vi "Actor Core.vi"(8 "error in":errorcluster, 11 "Agilent DSO-X 3032A in":refnum<class "Agilent DSO-X 3032A.lvclass">) -> (0 "error out":errorcluster, 3 "Actor out":refnum<class "Actor.lvclass">)   [LabVIEW 2014, in "Agilent DSO-X 3032A.lvclass"]
doc: "(<B>Filename</B>: Actor Framework.lvlib:Actor.lvclass:Actor Core.vi)\n\nReceives messages to the actor, reacts to them, and initiates any error handling that may shut the actor down.\n\nDescendant classes may override this VI to append parallel tasks for the actor to complete while it handles messages. Overrides use the Call Parent Method node."
uses:
  Agilent DSO-X 3032A.lvclass
  <vilib>/ActorFramework/Actor/Actor.lvclass
  Framework/Model/Data/Data1D/Data1D.lvclass
  Channel Settings.ctl
  Agilent DSO-X 3032A.lvclass/Agilent DSO-X 3032A.ctl
  <vilib>/ActorFramework/Actor/Actor.lvclass/Actor.ctl
  <vilib>/ActorFramework/Message Enqueuer/Message Enqueuer.lvclass/Message Enqueuer.ctl
  Framework/Interfaces/Pipelined Actor/Pipelined Actor Messages/Do Main Action Msg/Do Main Action Msg.lvclass/Do Main Action Msg.ctl
  Agilent DSO-X 3032A Messages/Write Instrument Handle Msg/Write Instrument Handle Msg.lvclass/Write Instrument Handle Msg.ctl
  Agilent DSO-X 3032A Messages/Read Config From Device Msg/Read Config From Device Msg.lvclass/Read Config From Device Msg.ctl
  Agilent DSO-X 3032A Messages/Write Timeout Msg/Write Timeout Msg.lvclass/Write Timeout Msg.ctl
  Agilent DSO-X 3032A Messages/Write Settings Msg/Write Settings Msg.lvclass/Write Settings Msg.ctl
  Agilent DSO-X 3032A Messages/Write CurrentChannel Msg/Write CurrentChannel Msg.lvclass/Write CurrentChannel Msg.ctl
  <vilib>/ActorFramework/Message Enqueuer/Init from Existing Queue.vi
  <vilib>/ActorFramework/Message Enqueuer/Enqueue.vi
  <vilib>/ActorFramework/Message Priority Queue/Priority Enqueue.vi
  <vilib>/ActorFramework/Message Enqueuer/Message Enqueuer.lvclass
  Framework/Model/Data/AbstractData/AbstractData.lvclass
  Framework/Interfaces/Pipelined Actor/Pipelined Actor Messages/Do Main Action Msg/Do Main Action Msg.lvclass
  Framework/Hardware/Device/Device Messages/Disconnect Msg/Disconnect Msg.lvclass
  Agilent DSO-X 3032A Messages/Write Instrument Handle Msg/Write Instrument Handle Msg.lvclass
  Agilent DSO-X 3032A Messages/Read Config From Device Msg/Read Config From Device Msg.lvclass
  Agilent DSO-X 3032A Messages/Write Timeout Msg/Write Timeout Msg.lvclass
  Agilent DSO-X 3032A Messages/Write Settings Msg/Write Settings Msg.lvclass
  Agilent DSO-X 3032A Messages/Write CurrentChannel Msg/Write CurrentChannel Msg.lvclass
  Framework/Hardware/ReadoutDevice/ReadoutDevice.lvclass
  Framework/Interfaces/Viewable Actor/Viewable Actor.lvclass
  Framework/Interfaces/Observable Actor/Observable Actor.lvclass
panel:
  in  "Channel":string(combo)="CHAN1"
  in  "Timeout, ms":i32=1000000
  in  "Channel Settings":T1={"Dt"=0.002, "#samples"=10000, "t0"=0.0} {"Dt" format="%.2e"}
  in  "Path":path
  out "isReading":bool
  out "Latest Data":refnum<class "Data1D.lvclass">
  in  "Save":bool
  in  "Resource name":refnum<k15>="AGILENT"
  in  "Disconnect":bool
  in  "Connect":bool
  in  "Read Conf":bool
  out "Stop":bool=TRUE
  in  "Read":bool
  out "Preview Graph":waveform(dbl)(graph)
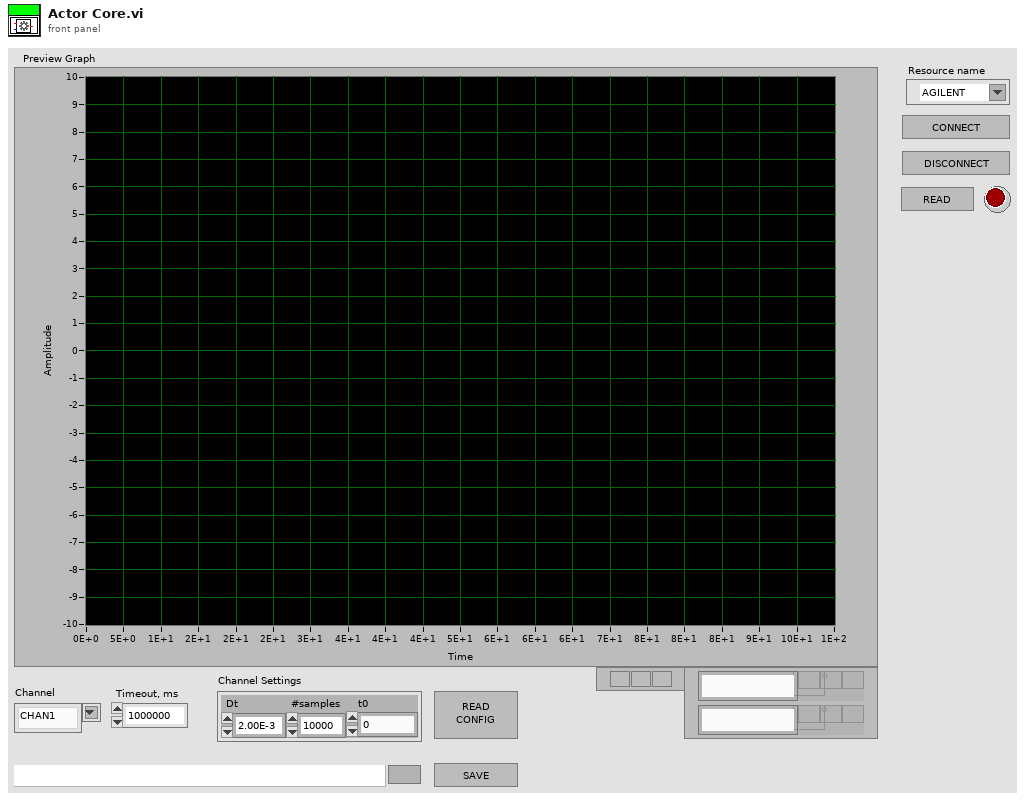
[diagram p1: front panel]
types:
  T1 = typedef "Agilent DSO-X 3032A.lvclass/Channel Settings.ctl" = cluster{"Dt":dbl, "#samples":i32, "t0":dbl}
  T2 = typedef "Observable Actor.lvlib/Observable Actor.lvclass/Observer.ctl" = refnum<queue>
  T3 = enum16{"open", "replace", "create", "open or create", "replace or create", "replace or create with confirmation"}
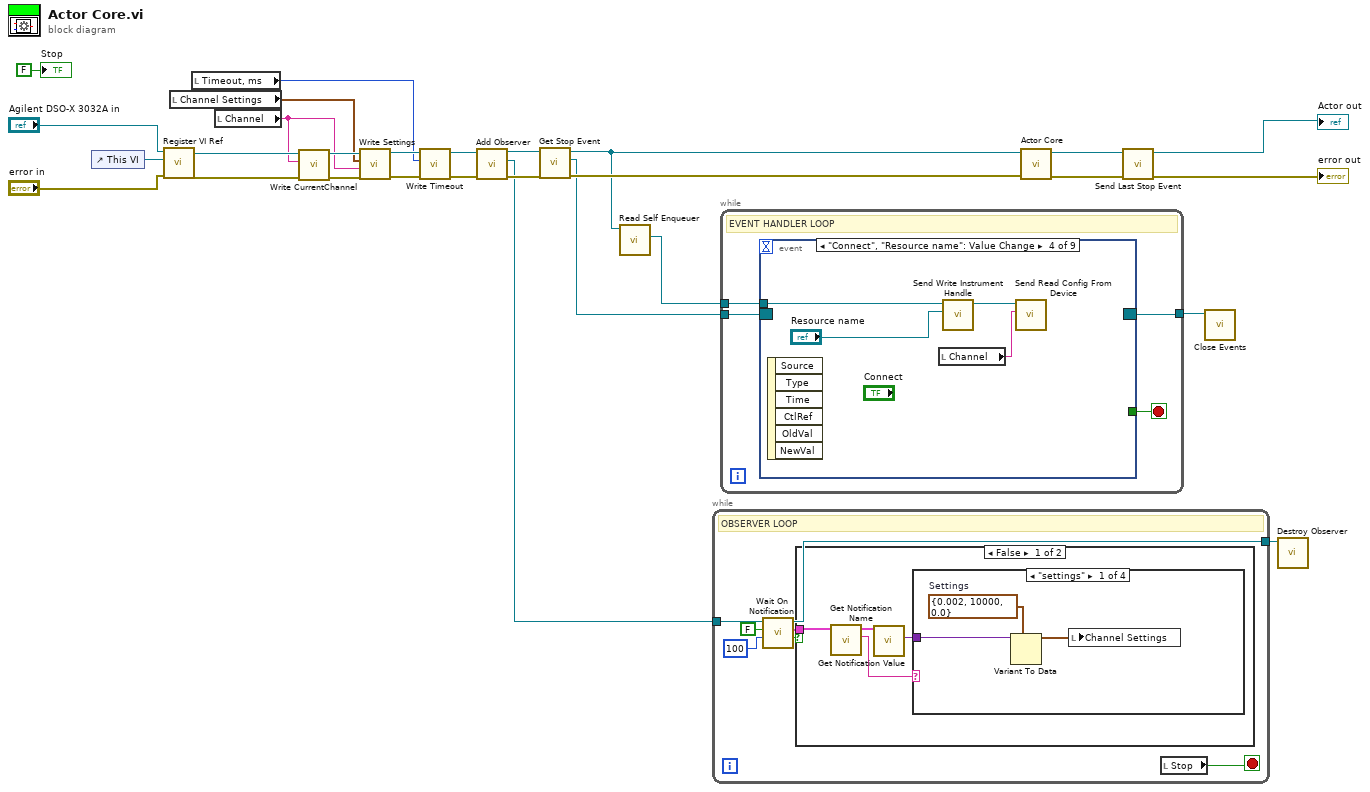
[diagram p0: block diagram]
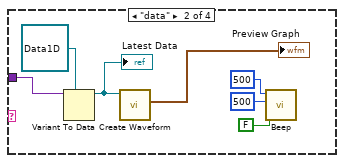
[diagram p2: hidden frame]
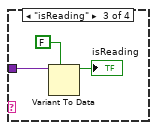
[diagram p3: hidden frame]
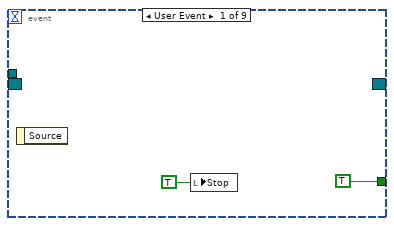
[diagram p6: hidden frame]
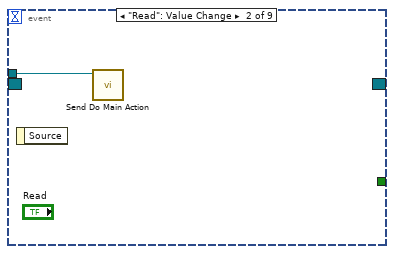
[diagram p7: hidden frame]
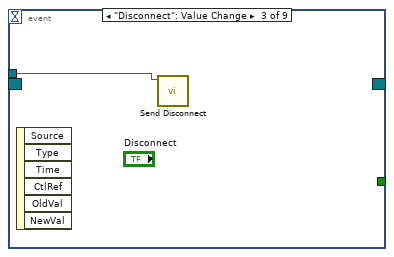
[diagram p8: hidden frame]
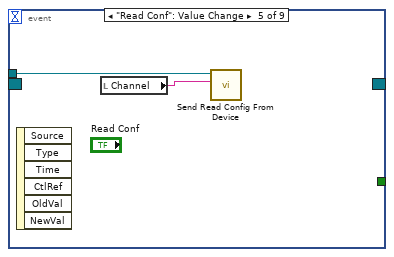
[diagram p9: hidden frame]
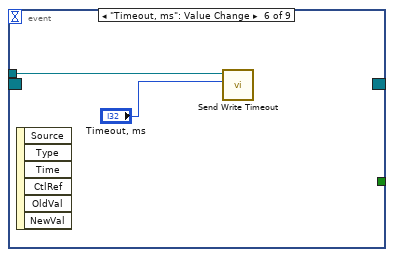
[diagram p10: hidden frame]
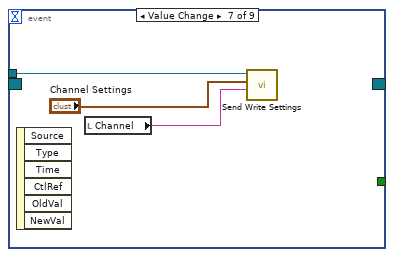
[diagram p11: hidden frame]
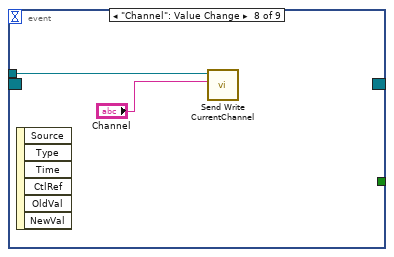
[diagram p12: hidden frame]
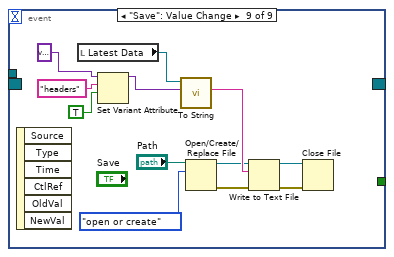
[diagram p13: hidden frame]
diagram:
  n1 = control-ref of="This VI"() -> (w27:refnum<vi>)
  n2 = call "Register VI Ref.vi"("error in (no error)"="error in", "VI ref"=w27, "Viewable Actor in"="Agilent DSO-X 3032A in") -> ("error out"=w10:errorcluster, "Viewable Actor out"=w11:refnum<class "Agilent DSO-X 3032A.lvclass">)  [unwired: 7 in]
  n3 = local read "Channel Settings"() -> (w7:T1)
  n4 = local read "Timeout, ms"() -> (w1:i32)
  n5 = local read "Channel"() -> (w8:string)
  n6 = call "Write CurrentChannel.vi"("error in (no error)"=w10, "CurrentChannel"=w8, "Agilent DSO-X 3032A in"=w11) -> ("error out"=w9:errorcluster, "Agilent DSO-X 3032A out"=w12:refnum<class "Agilent DSO-X 3032A.lvclass">)  [unwired: 7 in]
  n7 = call "Write Settings.vi"("error in (no error)"=w9, "Channel"=w8, "Settings"=w7, "Agilent DSO-X 3032A in"=w12) -> ("error out"=w4:errorcluster, "Agilent DSO-X 3032A out"=w5:refnum<class "Agilent DSO-X 3032A.lvclass">)  [unwired: 6 in]
  n8 = call "Write Timeout.vi"("error in (no error)"=w4, "Timeout"=w1, "Agilent DSO-X 3032A in"=w5) -> ("error out"=w3:errorcluster, "Agilent DSO-X 3032A out"=w2:refnum<class "Agilent DSO-X 3032A.lvclass">)  [unwired: 7 in]
  n9 = call-dynamic "Add Observer.vi"("error in (no error)"=w3, "Observable Actor in"=w2) -> ("error out"=w26:errorcluster, "new observer"=w24:T2, "Observable Actor out"=w23:refnum<class "Agilent DSO-X 3032A.lvclass">)  [unwired: 7 in]
  n10 = call-dynamic "Get Stop Event.vi"("error in (no error)"=w26, "Observable Actor in"=w23) -> ("error out"=w22:errorcluster, "Events"=w21:refnum<event-registration>, "Observable Actor out"=w13:refnum<class "Agilent DSO-X 3032A.lvclass">)  [unwired: 7 in]
  n11 = call <vilib>:"Read Self Enqueuer.vi"("Actor"=w13) -> ("Self Enqueuer"=w25:refnum<class "Message Enqueuer.lvclass">)  [unwired: 10 in]
  n12 = while {
    tunnel: w24 -> [w30]
    tunnel: [w29] -> w17
    stop <- w35 stop-if-true
    # "OBSERVER LOOP"
    n13 = call "Wait On Notification.vi"("timeout in ms (-1)"=100, "ignore previous (F)"=FALSE, "observer in"=w30) -> ("timed out?"=w31:bool, "notification"=w32:cluster{"value":variant, "name":string}, "observer out"=w29:T2)  [unwired: 5 in, 1 out]
    n14 = case shown="False" w31 {
      tunnel: w32 -> [w38 _]
      frame False {
        n15 = call "Get Notification Name.vi"("notification in"=w38) -> ("name"=w36:string, "notification out"=w37:cluster{"value":variant, "name":string})  [unwired: 9 in]
        n16 = call "Get Notification Value.vi"("notification in"=w37) -> ("data"=w39:variant)  [unwired: 7 in, 1 out]
        n17 = case shown="\"settings\"" w36 {
          tunnel: w39 -> [w42 w49 w51 _]
          frame "settings" {
            w41 = T1 {"Dt"=0.002, "#samples"=10000, "t0"=0.0}  # Settings
            n18 = Variant To Data(type=w41, Variant=w42) -> (data=w40:T1)  [unwired: 1 in, 1 out]
            n19 = local write "Channel Settings"(w40) -> ()
          }
          frame "data" {
            n20 = Variant To Data(type=refnum<class "Data1D.lvclass"> refnum ("Data1D in"), Variant=w49) -> (data=w47:refnum<class "Data1D.lvclass">)  [unwired: 1 in, 1 out]
            "Latest Data" <- w47
            n21 = call "Create Waveform.vi"("Data1D in"=w47) -> ("Waveform"=→"Preview Graph":waveform(dbl))  [unwired: 8 in, 2 out]
            n22 = call <vilib>:"Beep.vi"("use system alert? (T)"=FALSE, "duration (msec)"=u32 500, "frequency (Hz)"=u32 500) -> ()  [unwired: 9 in]
          }
          frame "isReading" {
            n23 = Variant To Data(type=FALSE, Variant=w51) -> (data=→"isReading":bool)  [unwired: 1 in, 1 out]
          }
          frame Default {
          }
        }
      }
      frame True {
      }
    }
    n24 = local read "Stop"() -> (w35:bool)
  }
  n25 = while {
    tunnel: w21 -> [w56]
    tunnel: w25 -> [w55]
    tunnel: [w54] -> w20
    stop <- w53 stop-if-true
    # "EVENT HANDLER LOOP"
    n26 = event shown="[3] \"Connect\", \"Resource name\": Value Change" {
      selector: w56 -> [_ _ _ _ _ _ _ _ _]
      dyn-events: [_ _ _ _ _ _ _ _ _] -> w54
      timeout: _ -> [_ _ _ _ _ _ _ _ _]
      tunnel: w55 -> [_ w59 w60 w64 w66 w68 w71 w73 _]
      tunnel: [TRUE _ _ _ _ _ _ _ _] -> w53
      event User Event {
        n27 = event-data() -> ()  [unwired: 1 in, 1 out]
        n28 = local write "Stop"(TRUE ("Stop")) -> ()
      }
      event "Read": Value Change {
        n29 = event-data() -> ()  [unwired: 1 in, 1 out]
        n30 = call "Send Do Main Action.vi"("Message Enqueuer"=w59) -> ()  [unwired: 9 in, 2 out]
      }
      event "Disconnect": Value Change {
        n31 = event-data() -> ()  [unwired: 1 in, 6 out]
        n32 = call "Send Disconnect.vi"("Message Enqueuer"=w60) -> ()  [unwired: 9 in, 2 out]
      }
      event "Connect", "Resource name": Value Change {
        n33 = event-data() -> ()  [unwired: 1 in, 6 out]
        n34 = local read "Channel"() -> (w62:string)
        n35 = call "Send Write Instrument Handle.vi"("Resource name"="Resource name", "Message Enqueuer"=w64) -> ("Message Enqueuer out"=w61:refnum<class "Message Enqueuer.lvclass">)  [unwired: 8 in, 1 out]
        n36 = call "Send Read Config From Device.vi"("Channel"=w62, "Message Enqueuer"=w61) -> ()  [unwired: 8 in, 2 out]
      }
      event "Read Conf": Value Change {
        n37 = event-data() -> ()  [unwired: 1 in, 6 out]
        n38 = local read "Channel"() -> (w65:string)
        n39 = call "Send Read Config From Device.vi"("Channel"=w65, "Message Enqueuer"=w66) -> ()  [unwired: 8 in, 2 out]
      }
      event "Timeout, ms": Value Change {
        n40 = event-data() -> ()  [unwired: 1 in, 6 out]
        n41 = call "Send Write Timeout.vi"("Timeout"="Timeout, ms", "Message Enqueuer"=w68) -> ()  [unwired: 8 in, 2 out]
      }
      event Value Change {
        n42 = event-data() -> ()  [unwired: 1 in, 6 out]
        n43 = local read "Channel"() -> (w69:string)
        n44 = call "Send Write Settings.vi"("Channel"=w69, "Settings"="Channel Settings", "Message Enqueuer"=w71) -> ()  [unwired: 7 in, 2 out]
      }
      event "Channel": Value Change {
        n45 = event-data() -> ()  [unwired: 1 in, 6 out]
        n46 = call "Send Write CurrentChannel.vi"("CurrentChannel"="Channel", "Message Enqueuer"=w73) -> ()  [unwired: 8 in, 2 out]
      }
      event "Save": Value Change {
        n47 = event-data() -> ()  [unwired: 1 in, 6 out]
        n48 = local read "Latest Data"() -> (w85:refnum<class "Data1D.lvclass">)
        n49 = Set Variant Attribute(Variant=variant ("variant"), name="headers", value=TRUE ("Save to single file")) -> (Variant out=w76:variant)  [unwired: 1 in, 2 out]
        n50 = call-dynamic "To String.vi"("Parameters"=w76, "Data1D in"=w85) -> ("String"=w84:string)  [unwired: 7 in, 2 out]
        n51 = Open/Create/Replace File(file path (use dialog)="Path", operation (0:open)=T3."open or create") -> (refnum out=w83:refnum<file>, error out=w81:errorcluster)  [unwired: 4 in, 1 out]
        n52 = Write to Text File(file (use dialog)=w83, text=w84, error in=w81) -> (refnum out=w82:refnum<file>, error out=w80:errorcluster)  [unwired: 1 in, 1 out]
        n53 = Close File(refnum=w82, error in=w80) -> ()  [unwired: 2 out]
      }
    }
  }
  n54 = call-parent "Actor Core.vi"("error in"=w22, "Actor in"=w13) -> ("error out"=w18:errorcluster, "Actor out"=w19:refnum<class "Actor.lvclass">)  [unwired: 8 in]
  n55 = call "Send Last Stop Event.vi"("error in (no error)"=w18, "Actor in"=w19) -> ("error out"=→"error out":errorcluster, "Actor  out"=→"Actor out":refnum<class "Actor.lvclass">)  [unwired: 8 in]
  n56 = call "Close Events.vi"("events"=w20) -> ()  [unwired: 11 in]
  n57 = call "Destroy Observer.vi"("observer in"=w17) -> ()  [unwired: 11 in]
  "Stop" <- FALSE ("Stop")
